vi "Init Interface.vi"(8 "error in":errorcluster, 9 "Config Section":string, 10 "hse-config":refnum<class "config-base.lvclass">, 11 "DB-MySQL":refnum<class "DB-MySQL.lvclass">) -> (0 "error out":errorcluster, 3 "DB-MySQL":refnum<class "DB-MySQL.lvclass">)   [LabVIEW 2020, in "hse-db-mysql.lvlib" / "DB-MySQL.lvclass"]
doc: "____\nHAMPEL SOFTWARE ENGINEERING v1.4.0 (2023-12-19 09:52)"
uses:
  DB-MySQL.lvclass
  hse-libraries/Source/hse-configuration/config-base/config-base.lvclass
  DB-MySQL.lvclass/DB-MySQL.ctl
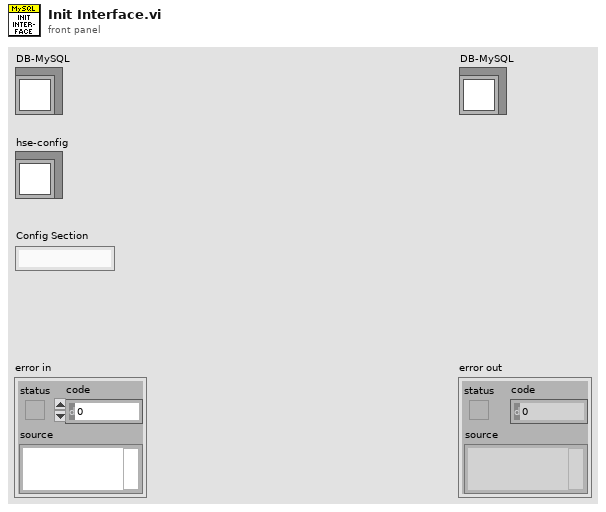
[diagram p1: front panel]
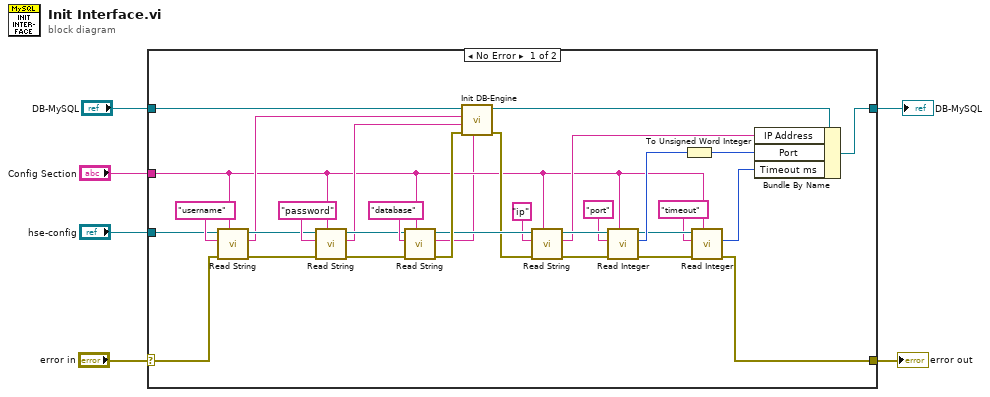
[diagram p0: block diagram]
diagram:
  n1 = case shown="No Error" "error in" {
    selector: "error in" -> [w37 w39]
    tunnel: [w8 w39] -> w5
    tunnel: [w23 w38] -> w1
    tunnel: "DB-MySQL" -> [w35 w38]
    tunnel: "hse-config" -> [w27 _]
    tunnel: "Config Section" -> [w11 _]
    frame No Error {
      n2 = call-dynamic "Read String.vi"("Section"=w11, "error in"=w37, "Key"="username", "config-base in"=w27) -> ("error out"=w28:errorcluster, "Value"=w26:string, "config-base out"=w29:refnum<class "config-base.lvclass">)  [unwired: 5 in]
      n3 = call-dynamic "Read String.vi"("Section"=w11, "error in"=w28, "Key"="password", "config-base in"=w29) -> ("error out"=w32:errorcluster, "Value"=w25:string, "config-base out"=w33:refnum<class "config-base.lvclass">)  [unwired: 5 in]
      n4 = call-dynamic "Read String.vi"("Section"=w11, "error in"=w32, "Key"="database", "config-base in"=w33) -> ("error out"=w36:errorcluster, "Value"=w7:string, "config-base out"=w22:refnum<class "config-base.lvclass">)  [unwired: 5 in]
      n5 = call-dynamic "Init DB-Engine.vi"("Database"=w7, "error in"=w36, "Password"=w25, "User"=w26, "DB-Engine in"=w35) -> ("error out"=w21:errorcluster, "DB-Engine out"=w24:refnum<class "DB-MySQL.lvclass">)  [unwired: 5 in]
      n6 = call-dynamic "Read String.vi"("Section"=w11, "error in"=w21, "Key"="ip", "config-base in"=w22) -> ("error out"=w19:errorcluster, "Value"=w17:string, "config-base out"=w18:refnum<class "config-base.lvclass">)  [unwired: 5 in]
      n7 = call-dynamic "Read Integer.vi"("Section"=w11, "error in"=w19, "Key"="port", "config-base in"=w18) -> ("error out"=w13:errorcluster, "Value"=w15:i64, "config-base out"=w12:refnum<class "config-base.lvclass">)  [unwired: 5 in]
      n8 = To Unsigned Word Integer(number=w15) -> (unsigned 16bit integer=w14:u16)
      n9 = call-dynamic "Read Integer.vi"("Section"=w11, "error in"=w13, "Key"="timeout", "config-base in"=w12) -> ("error out"=w8:errorcluster, "Value"=w9:i64)  [unwired: 5 in, 1 out]
      n10 = Bundle By Name(cluster=w24, "IP Address"=w17, "Port"=w14, "Timeout ms"=w9) -> (w23:refnum<class "DB-MySQL.lvclass">)
    }
    frame Error {
    }
  }
  "error out" <- w5
  "DB-MySQL" <- w1
